vi "Create_Default_Destinations.vi"(8 "error in (no error)":errorcluster, 9 "Destination Name":string, 10 "Destination Path":path, 11 "AB_WebService in":refnum<class "AB_WebService.lvclass">) -> (0 "error out":errorcluster, 2 "default dests":refnum<class "AB_Destination.lvclass">[](array[class]), 3 "AB_WebService out":refnum<class "AB_WebService.lvclass">)   [LabVIEW 2020, in "AB_WebService.lvclass"]
uses:
  <vilib>/AppBuilder/AB_Classes/WebService/AB_WebService.lvclass
  <vilib>/AppBuilder/AB_Classes/Destination/AB_Destination.lvclass
  <resource>/Framework/Providers/Common/provcom_StringGlobals.vi
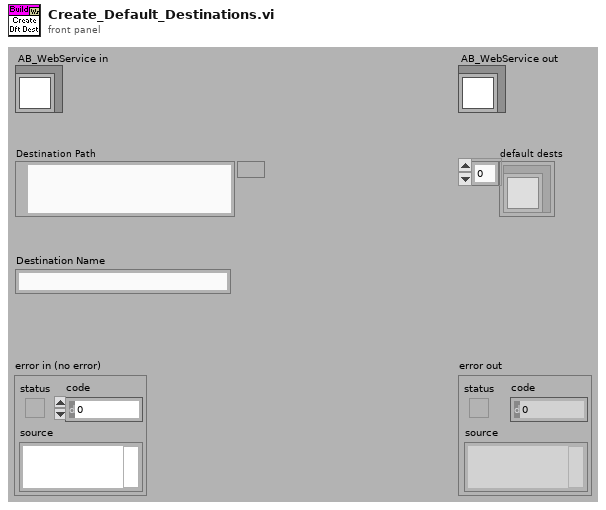
[diagram p1: front panel]
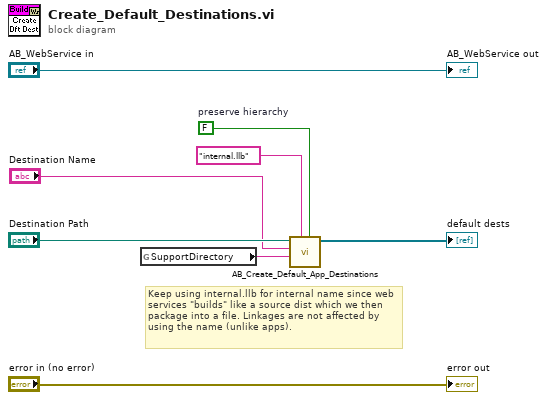
[diagram p0: block diagram]
diagram:
  w1 = FALSE  # preserve hierarchy
  # "Keep using internal.llb for internal name since web services \"builds\" like a source dist which we then package into a file. Linkages are not affected by using the name (unlike apps)."
  n1 = global read "provcom_StringGlobals.vi" "SupportDirectory"() -> (w7:string)
  n2 = call <vilib>:"AB_Create_Default_App_Destinations.vi"("preserve hierarchy (T)"=w1, "internal dir name"="internal.llb", "SupportDirectory"=w7, "App Name"="Destination Name", "App Destination Path"="Destination Path") -> ("default app dests"=→"default dests":refnum<class "AB_Destination.lvclass">[])  [unwired: 1 in, 5 out]
  "error out" <- "error in (no error)"
  "AB_WebService out" <- "AB_WebService in"
